vi "Init.vi"(8 "error in (no error)":errorcluster, 11 "Instrument in":refnum<class "Instrument.lvclass">) -> (0 "error out":errorcluster, 3 "Instrument out":refnum<class "Instrument.lvclass">)   [LabVIEW 2018, in "Instrument.lvclass"]
uses:
  Instrument.lvclass
  Instrument.lvclass/Instrument.ctl
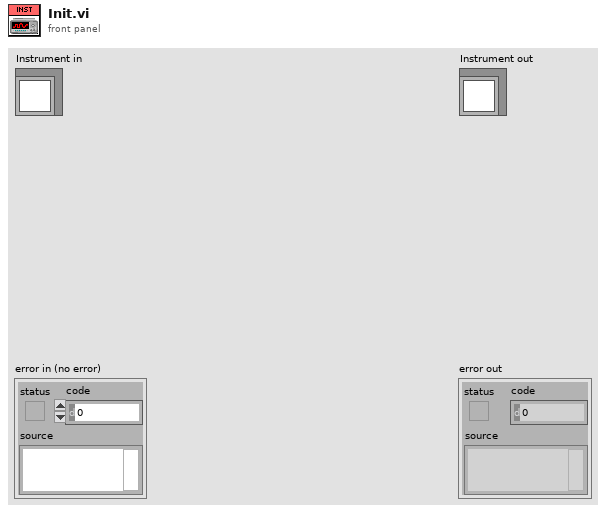
[diagram p1: front panel]
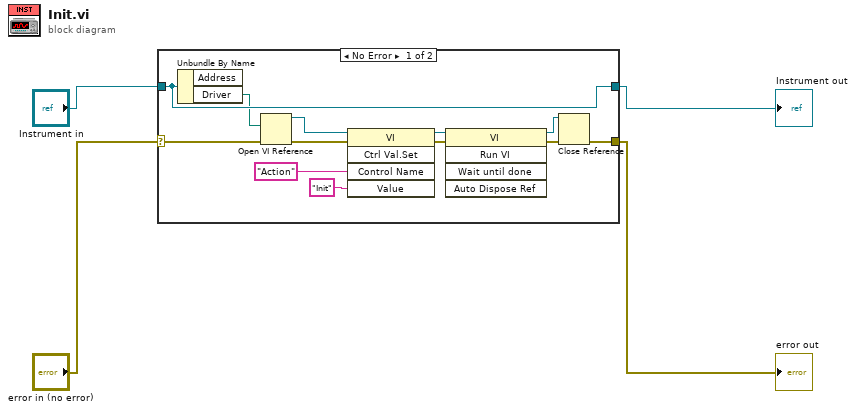
[diagram p0: block diagram]
diagram:
  n1 = case shown="No Error" "error in (no error)" {
    selector: "error in (no error)" -> [w11 w18]
    tunnel: [w10 w18] -> w3
    tunnel: [w16 w17] -> w1
    tunnel: "Instrument in" -> [w16 w17]
    frame No Error {
      n2 = Unbundle By Name(w16) -> ("Driver"=w15:path)  [unwired: 1 out]
      n3 = Open VI Reference(vi path=w15, error in (no error)=w11) -> (vi reference=w14:refnum<vi>, error out=w9:errorcluster)  [unwired: 4 in]
      n4 = invoke class="VI" method="Ctrl Val.Set"(reference=w14, error in=w9, "Control Name"="Action", "Value"="Init" ("Control Name")) -> (reference out=w7:refnum<vi>, error out=w8:errorcluster)  [unwired: 1 in, 3 out]
      n5 = invoke class="VI" method="Run VI"(reference=w7, error in=w8) -> (reference out=w6:refnum<vi>, error out=w5:errorcluster)  [unwired: 3 in, 3 out]
      n6 = Close Reference(reference=w6, error in (no error)=w5) -> (error out=w10:errorcluster)
    }
    frame Error {
    }
  }
  "error out" <- w3
  "Instrument out" <- w1
